vi "loads_builder_antigo.vi"(7 "measure?":dbl, 10 "Load (pu)":string, 11 "Loads data":path) -> (3 "Loads (out)":string)   [LabVIEW 2019]
uses:
  <vilib>/Utility/file.llb/Read From Spreadsheet File (DBL).vi
panel:
  in  "Frequency (Hz)":dbl=50.0
  in  "Font (Vrms)":dbl=4160.0
  out "Powers":dbl[][](array[numeric])
  out "nós":dbl[](array[numeric])
  # "LOADS BUILDER"
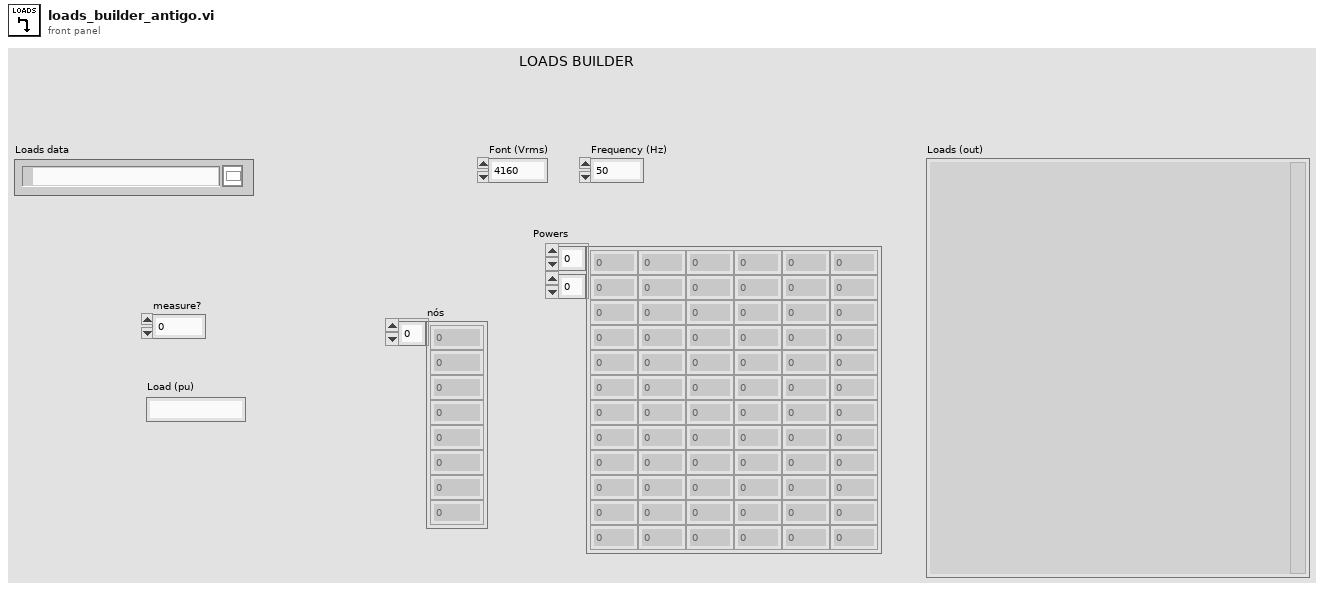
[diagram p1: front panel]
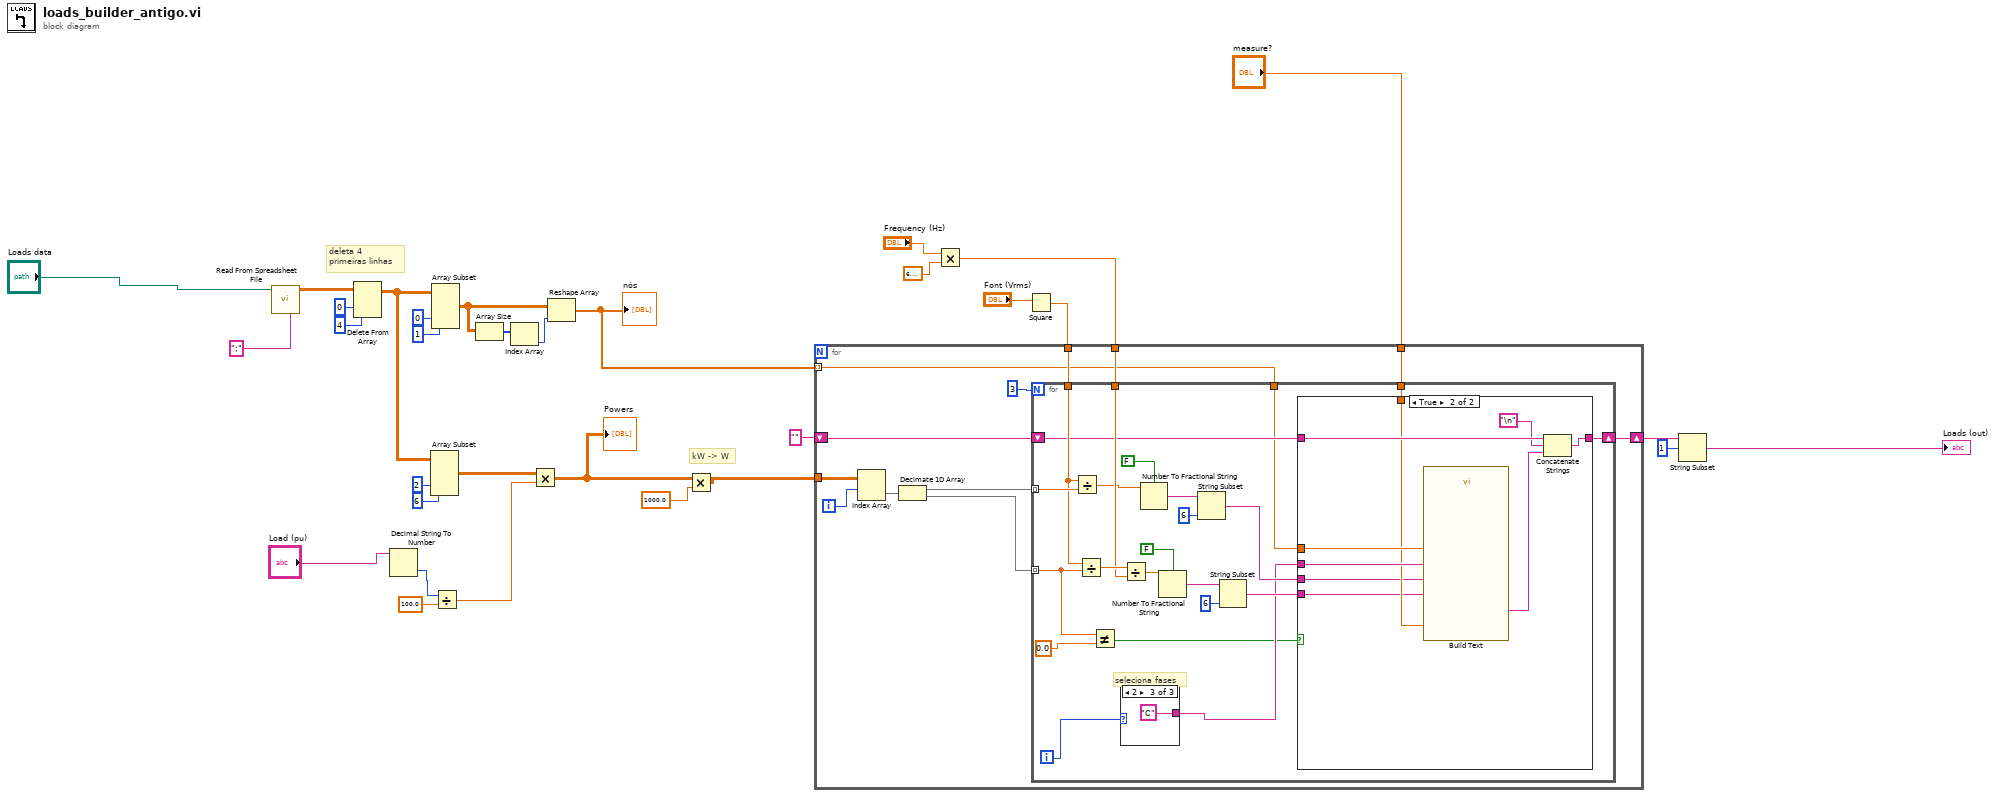
[diagram p0: block diagram]
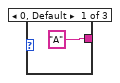
[diagram p3: hidden frame]
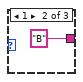
[diagram p4: hidden frame]
diagram:
  # "kW -> W"
  # "deleta 4\nprimeiras linhas"
  n1 = call-poly <vilib>:"Read From Spreadsheet File.vi"("delimiter (\\t)"=";" ("delimiter (\\t)"), "file path (dialog if empty)"="Loads data") -> ("all rows"=w29:dbl[][])  [unwired: 5 in, 4 out]
  n2 = Delete From Array(array=w29, length=4, index (row)=0) -> (array with subset deleted=w20:dbl[][])  [unwired: 1 in, 1 out]
  n3 = Decimal String To Number(string="Load (pu)") -> (number=w2:i32)  [unwired: 2 in, 1 out]
  n4 = Array Subset(array=w20, index (col)=2 ("index"), length (col)=6 ("length")) -> (w14:dbl[][])  [unwired: 2 in]
  n5 = Array Subset(array=w20, index (col)=0 ("index"), length (col)=1 ("length")) -> (w26:dbl[][])  [unwired: 2 in]
  n6 = Divide(x=w2, y=100.0) -> (x/y=w1:dbl)
  n7 = Array Size(array=w26) -> (size(s)=w25:i32[])
  n8 = Index Array(array=w25) -> (element=w24:i32)  [unwired: 1 in]
  n9 = Multiply(x=w14, y=w1) -> (x*y=w5:dbl[][])
  "Powers" <- w5
  n10 = Reshape Array(w26, w24) -> (w23:dbl[])
  "nós" <- w23
  n11 = Multiply(x=w5, y=1000.0) -> (x*y=w7:dbl[][])
  n12 = Multiply(x="Frequency (Hz)", y=6.283185307179586) -> (x*y=w15:dbl)
  n13 = Square(x="Font (Vrms)") -> (x^2=w18:dbl)
  n14 = for {
    tunnel: w23 -> [w36] mode=indexing
    tunnel: w7 -> [w44]
    tunnel: w18 -> [w38]
    tunnel: w15 -> [w37]
    shift-right: [w34] -> w12
    shift-left: "" -> [w35]
    tunnel: "measure?" -> [w33]
    i -> [w43]
    n15 = Index Array(array=w44, index (row)=w43) -> (element=w41:dbl[])  [unwired: 1 in]
    n16 = Decimate 1D Array(w41) -> (w40:dbl[], w39:dbl[])
    n17 = for {
      N: 3 -> [_]
      tunnel: w40 -> [w67] mode=indexing
      tunnel: w39 -> [w56] mode=indexing
      tunnel: w38 -> [w66]
      tunnel: w37 -> [w64]
      tunnel: w36 -> [w50]
      shift-right: [w54] -> w34
      shift-left: w35 -> [w55]
      tunnel: w33 -> [w45]
      i -> [w57]
      # "seleciona fases"
      n18 = Divide(x=w66, y=w67) -> (x/y=w63:dbl)
      n19 = Divide(x=w66, y=w56) -> (x/y=w65:dbl)
      n20 = Not Equal?(x=w56, y=0.0 ("x")) -> (x != y?=w49:bool)
      n21 = case shown="2" w57 {
        tunnel: ["A" "B" "C"] -> w51
        frame 0, Default {
        }
        frame 1 {
        }
        frame 2 {
        }
      }
      n22 = Divide(x=w65, y=w64) -> (x/y=w62:dbl)
      n23 = Number To Fractional String(use system decimal point (T)=FALSE, number=w63) -> (F-format string=w61:string)  [unwired: 2 in]
      n24 = Number To Fractional String(use system decimal point (T)=FALSE, number=w62) -> (F-format string=w59:string)  [unwired: 2 in]
      n25 = String Subset(string=w61, length (rest)=6 ("length (rest)")) -> (substring=w52:string)  [unwired: 1 in]
      n26 = String Subset(string=w59, length (rest)=6 ("length (rest)")) -> (substring=w53:string)  [unwired: 1 in]
      n27 = case shown="True" w49 {
        tunnel: w55 -> [w68 w77]
        tunnel: [w68 w74] -> w54
        tunnel: w53 -> [_ w70]
        tunnel: w52 -> [_ w69]
        tunnel: w51 -> [_ w73]
        tunnel: w50 -> [_ w72]
        tunnel: w45 -> [_ w71]
        frame False {
        }
        frame True {
          n28 = call "Build Text"("reatancia"=w70, "no"=w72, "fase"=w73, "resistencia"=w69, "measure"=w71) -> ("Result"=w75:string)  [unwired: 9 in, 1 out]
          n29 = Concatenate Strings(w77, "\n", w75) -> (w74:string)
        }
      }
    }
  }
  n30 = String Subset(string=w12, offset (0)=1) -> (substring=→"Loads (out)":string)  [unwired: 1 in]
